vi "stepper driver -- void.vi"(6 "Instrument Address":refnum<visa-resource-name>="ASRL3::INSTR", 7 "stepper driver action":T3=enum."stop", 10 "speed IN":dbl=0.23, 11 "number":dbl=2000.0 format="%#_13g") -> (1 "stepper motor state OUT":T2, 2 "speed":dbl, 3 "number out":dbl)   [LabVIEW 2019]
uses:
  stepper driver action.ctl
  stepper motor state.ctl
  internal stepper driver state -- BLM.ctl
panel:
  out "internal stepper driver state BLM OUT":T1={"initialized?"=TRUE, "VISA address"="GPIB0::25::INSTR", "stepper motor state"=enum."stopped", "Motor Address"="0", "speed"=0.0, "steps/rot"=8000.0, "vert increment"=0.0042, "target position"=2000.0, "mode"=enum."absolute", "current position"=0.0}
  in  "internal stepper driver state BLM":T1={"initialized?"=TRUE, "VISA address"="GPIB0::25::INSTR", "stepper motor state"=enum."stopped", "Motor Address"="0", "speed"=0.0, "steps/rot"=8000.0, "vert increment"=0.0042, "target position"=0.0, "mode"=enum."absolute", "current position"=0.0}
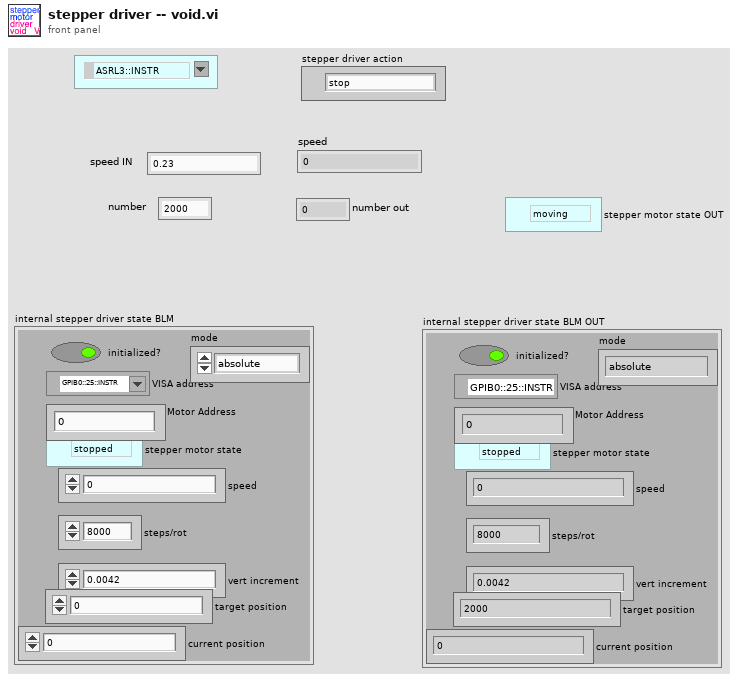
[diagram p1: front panel]
types:
  T1 = typedef "internal stepper driver state -- BLM.ctl" = cluster{"initialized?":bool, "VISA address":refnum<visa-resource-name>, "stepper motor state":T2, "Motor Address":string, "speed":dbl, "steps/rot":dbl, "vert increment":dbl, "target position":dbl, "mode":enum16{"absolute", "relative"}, "current position":dbl}
  T2 = typedef "stepper motor state.ctl" = enum16{"moving", "stopped"}
  T3 = typedef "stepper driver action.ctl" = enum16{"go", "void", "stop", "check", "init", "sync", "set", "set speed", "--check status", "--check value", "--handshake"}
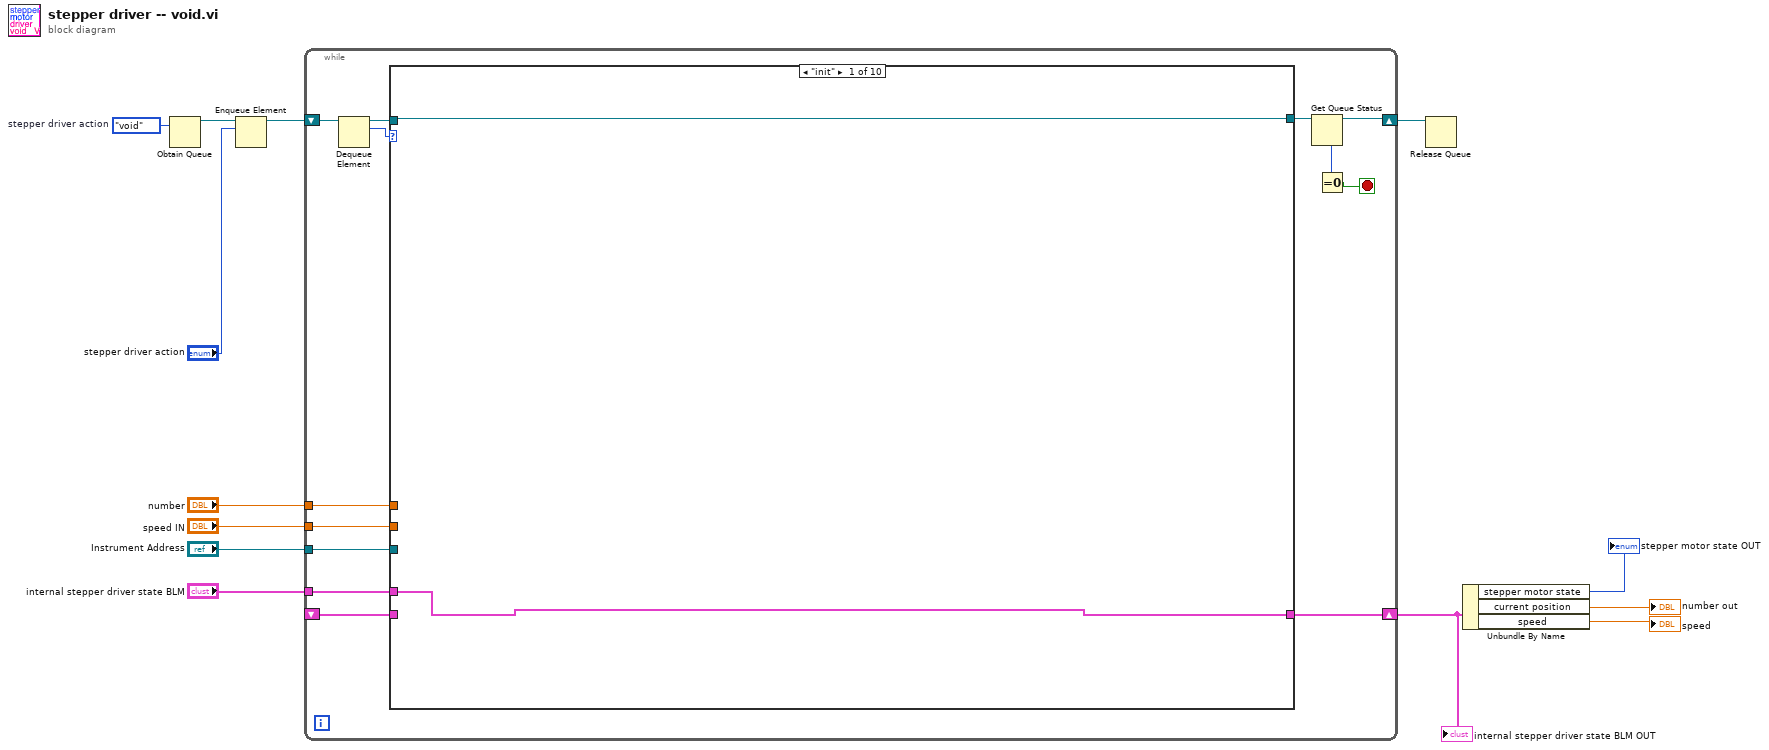
[diagram p0: block diagram]
diagram:
  w5 = stepper_driver_action."void"  # stepper driver action
  n1 = Obtain Queue(element data type=w5) -> (queue out=w4:refnum<queue>)  [unwired: 4 in, 2 out]
  n2 = Enqueue Element(queue=w4, element="stepper driver action") -> (queue out=w3:refnum<queue>)  [unwired: 2 in, 2 out]
  n3 = while {
    shift-right: [w26] -> w11
    shift-left: _ -> [w25]
    shift-right: [w18] -> w1
    shift-left: w3 -> [w17]
    tunnel: "internal stepper driver state BLM" -> [w24]
    tunnel: "number" -> [w23]
    tunnel: "Instrument Address" -> [w22]
    tunnel: "speed IN" -> [w21]
    stop <- w14 stop-if-true
    n4 = Dequeue Element(queue=w17) -> (queue out=w20:refnum<queue>, element=w16:T3)  [unwired: 2 in, 2 out]
    n5 = case shown="\"init\"" w16 {
      tunnel: [w28 w29 w31 w34 w35 w37 w39 w41 w43 w45] -> w26
      tunnel: w25 -> [_ w29 w31 w34 w35 w37 w39 w41 w43 w45]
      tunnel: [w27 w30 w32 w33 w36 w38 w40 w42 w44 w46] -> w19
      tunnel: w20 -> [w27 w30 w32 w33 w36 w38 w40 w42 w44 w46]
      tunnel: w24 -> [w28 _ _ _ _ _ _ _ _ _]
      tunnel: w23 -> [_ _ _ _ _ _ _ _ _ _]
      tunnel: w22 -> [_ _ _ _ _ _ _ _ _ _]
      tunnel: w21 -> [_ _ _ _ _ _ _ _ _ _]
      frame "init" {
      }
      frame "set" {
      }
      frame "set speed" {
        # "SPEED (rot/sec)\nincrement .0042"
      }
      frame "check", Default {
      }
      frame "--check status" {
      }
      frame "--check value" {
      }
      frame "void" {
      }
      frame "sync" {
      }
      frame "go" {
      }
      frame "stop" {
        # "SPEED (rot/sec)\nincrement .0042"
      }
    }
    n6 = Get Queue Status(queue=w19) -> (queue out=w18:refnum<queue>, # elements in queue=w15:i32)  [unwired: 2 in, 6 out]
    n7 = Equal To 0?(x=w15) -> (x = 0?=w14:bool)
  }
  "internal stepper driver state BLM OUT" <- w11
  n8 = Release Queue(queue=w1) -> ()  [unwired: 2 in, 3 out]
  n9 = Unbundle By Name(w11) -> ("stepper motor state"=→"stepper motor state OUT":T2, "current position"=→"number out":dbl, "speed"=→"speed":dbl)
